vi "UpdateToolbar.vi"(1 "ToolbarButtons":T1[](array[typedef]), 5 "error in (no error)":errorcluster) -> (19 "error out":errorcluster)   [LabVIEW 2014, in "UmlEditor.lvclass"]
uses:
  <resource>/Framework/Providers/Open_GDS/UML/UmlEditor_class/UmlEditor.lvclass
  <resource>/Framework/Providers/Open_GDS/UML/Graph_class/ToolbarButtonType.ctl
  <resource>/Framework/Providers/Open_GDS/UML/UMLEditor/UMLEditor tooltype.ctl
  <resource>/Framework/Providers/Open_GDS/UML/Graph_class/Graph.lvclass
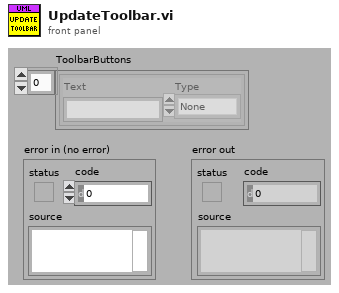
[diagram p1: front panel]
types:
  T1 = typedef "Graph.lvclass/ToolbarButtonType.ctl" = cluster{"Text":string, "Type":T2}
  T2 = typedef "UMLEditor tooltype.ctl" = enum16{"None", "Node", "Edge"}
  T3 = typedef "UmlEditor.lvclass/ObjectAttributes.ctl" = cluster{"ListeningQueueIn":refnum<queue>, "Event":refnum<user-event>, "UseProjectFolderAsBasePath":bool, "TypeSyncOption":bool, "Attr":string[], "ToolTip":cluster{"ToolTipOpen":bool, "LastToolTip":i32}, "ClassesToIgnore":string[], "UndoSize":i32, "OpenLastSavedFileWhenStarting":bool, "SyncOption":T4, "SyncTime(s)":i32, "Params":cluster{"IniParams":T5, "Value":string}[], "GraphButtons":refnum<vi>}
  T4 = typedef "UMLEditor_SyncOptions.ctl" = cluster{"IgnoreInstrLib":bool, "IgnoreUserLib":bool, "IgnoreViLib":bool}
  T5 = typedef "UmlEditor.lvclass/IniParamsType.ctl" = enum16{"I have problem with UML stability on my computer"}
  T6 = cluster{"left":i16, "top":i16, "right":i16, "bottom":i16}
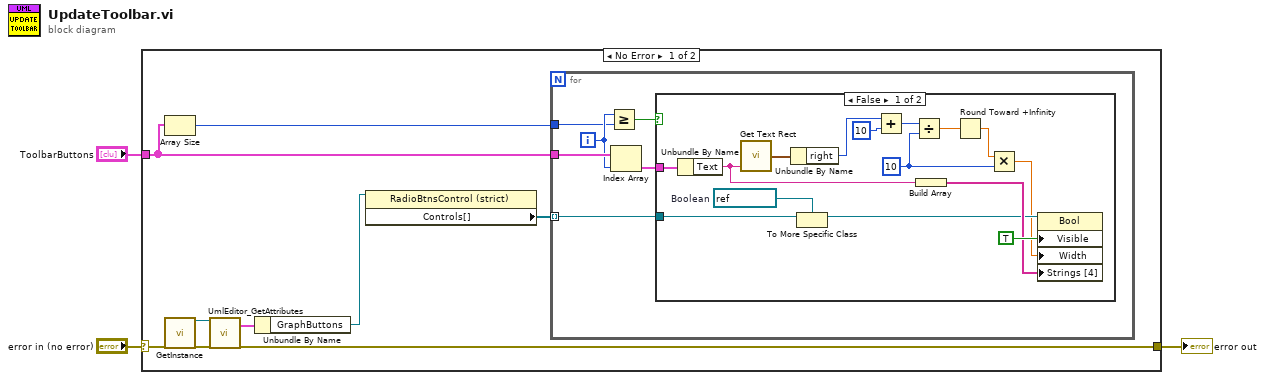
[diagram p0: block diagram]
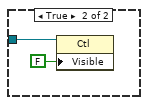
[diagram p2: hidden frame]
diagram:
  n1 = case shown="No Error" "error in (no error)" {
    selector: "error in (no error)" -> [w8 w36]
    tunnel: [w11 w36] -> w2
    tunnel: "ToolbarButtons" -> [w5 _]
    frame No Error {
      n2 = Array Size(array=w5) -> (size(s)=w4:i32)
      n3 = call <resource>:"GetInstance.vi"("error in (no error)"=w8) -> ("reference out"=w10:refnum<class "UmlEditor.lvclass">, "error out"=w9:errorcluster)  [unwired: 17 out]
      n4 = call <resource>:"UmlEditor_GetAttributes.vi"("reference in"=w10, "error in (no error)"=w9) -> ("Data"=w12:T3, "error out"=w11:errorcluster)  [unwired: 14 in, 2 out]
      n5 = Unbundle By Name(w12) -> ("GraphButtons"=w7:refnum<vi>)
      n6 = property class="RadioBtnsControl (strict)"(reference=w7) -> ("Controls[]"=w6:refnum<vi>[])  [unwired: 1 in, 2 out]
      n7 = for {
        tunnel: w6 -> [w14] mode=indexing
        tunnel: w5 -> [w18]
        tunnel: w4 -> [w16]
        i -> [w17]
        n8 = Greater Or Equal?(x=w17, y=w16) -> (x >= y?=w15:bool)
        n9 = Index Array(array=w18, index=w17) -> (element=w13:T1)
        n10 = case shown="False" w15 {
          tunnel: w14 -> [w21 w35]
          tunnel: w13 -> [w31 _]
          frame False {
            w22 = refnum<vi> refnum  # Boolean
            w24 = i16 10 ("y")
            n11 = Unbundle By Name(w31) -> ("Text"=w29:string)
            n12 = call <vilib>:"Get Text Rect.vi"("text"=w29) -> ("rect"=w30:T6)  [unwired: 8 in]
            n13 = Unbundle By Name(w30) -> ("right"=w28:i16)
            n14 = To More Specific Class(target class=w22, reference=w21) -> (specific class reference=w20:refnum<vi>)  [unwired: 1 in, 1 out]
            n15 = Add(x=w28, y=i16 10) -> (x+y=w26:i16)
            n16 = Divide(x=w26, y=w24) -> (x/y=w25:dbl)
            n17 = Build Array(w29) -> (w32:string[])
            n18 = Round Toward +Infinity(x=w25) -> (ceil(x): smallest int >= x=w23:dbl)
            n19 = Multiply(x=w23, y=w24) -> (x*y=w19:dbl)
            n20 = property class="Bool"(reference=w20, "Visible"=TRUE, "Width"=w19, "Strings [4]"=w32) -> ()  [unwired: 1 in, 2 out]
          }
          frame True {
            n21 = property class="Ctl"(reference=w35, "Visible"=FALSE) -> ()  [unwired: 1 in, 2 out]
          }
        }
      }
    }
    frame Error {
    }
  }
  "error out" <- w2
